vi "Start Connection Monitor.vi"(8 "error in (no error)":errorcluster, 10 "Configure":T1, 11 "RemoteControl.STM in":refnum<class "RemoteControl.STM.lvclass">) -> (0 "error out":errorcluster, 3 "RemoteControl.STM out":refnum<class "RemoteControl.STM.lvclass">)   [LabVIEW 2016, in "RemoteControl.STM.lvclass"]
uses:
  RemoteControl.STM.lvclass
  RemoteControl/Typedefs/PrivateEvents--RemoteControl.Configure.ctl
  RemoteControl/RemoteControl.lvclass
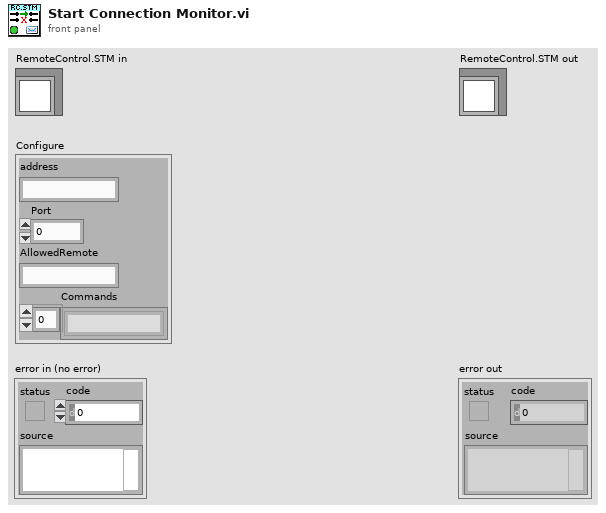
[diagram p1: front panel]
types:
  T1 = typedef "RemoteControl.lvclass/PrivateEvents--RemoteControl.Configure.ctl" = cluster{"address":string, "Port":u16, "AllowedRemote":string, "Commands":string[]}
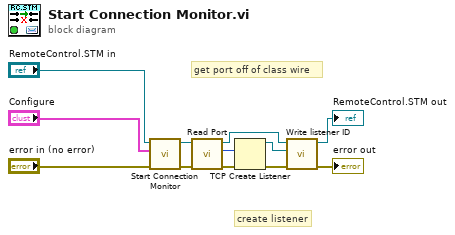
[diagram p0: block diagram]
diagram:
  # "get port off of class wire"
  # "create listener"
  n1 = call-parent "Start Connection Monitor.vi"("error in (no error)"="error in (no error)", "Configure"="Configure", "RemoteControl in"="RemoteControl.STM in") -> ("error out"=w1:errorcluster, "RemoteControl out"=w4:refnum<class "RemoteControl.STM.lvclass">)  [unwired: 7 in]
  n2 = call-dynamic "Read Port.vi"("error in (no error)"=w1, "RemoteControl in"=w4) -> ("error out"=w9:errorcluster, "Port"=w8:u16, "RemoteControl out"=w5:refnum<class "RemoteControl.STM.lvclass">)  [unwired: 7 in]
  n3 = TCP Create Listener(8:w9, 10:w8) -> (0:w6:errorcluster, 3:w7:refnum<k5>)  [unwired: 3 in, 1 out]
  n4 = call-dynamic "Write listener ID.vi"("error in (no error)"=w6, "listener ID"=w7, "RemoteControl.STM in"=w5) -> ("error out"=→"error out":errorcluster, "RemoteControl.STM out"=→"RemoteControl.STM out":refnum<class "RemoteControl.STM.lvclass">)  [unwired: 7 in]
